vi "Dashboard Main.vi"() -> ()   [LabVIEW 2020]
uses:
  <vilib>/Rock Robotics/Network Tables/NT Read Numeric Array.vi
  <vilib>/Rock Robotics/Network Tables/NT Read String.vi
  <vilib>/Rock Robotics/Network Tables/NT Read Number.vi
  <vilib>/Rock Robotics/Network Tables/NT Read Boolean.vi
  <vilib>/Rock Robotics/Network Tables/NT Write Number.vi
  <vilib>/Rock Robotics/Network Tables/NT Write Boolean.vi
panel:
  out "Popcorn Engaged":bool
  out "Camera Image 5":T1(plugin-control)
  in  "Camera Settings Right":T2={"Frame Rate"=30, "Compression"=30, "Size"=1, "DB Camera Config"=FALSE} {"Frame Rate" scale=1.0..30.0; "Compression" scale=100.0..-1.0; "Size" items=["640x480", "320x240", "160x120"]}
  in  "Camera Name Right":string(combo)="No Camera Selection"
  out "Camera Perf":string
  in  "Camera Settings":T2={"Frame Rate"=30, "Compression"=30, "Size"=1, "DB Camera Config"=FALSE} {"Frame Rate" scale=1.0..30.0; "Compression" scale=100.0..-1.0; "Size" items=["640x480", "320x240", "160x120"]}
  in  "TCP":refnum<k5>
  out "Robot IP":string
  in  "Dashboard Tab":T3(tab)
  in  "ARE YOU READY TO RUMBLE":bool
  out "Climb Override":bool
  out "Climbing Stages":sgl(slide) scale=0.0..10.0 scale format="%#_6p"
  out "Lidar":dbl(knob) scale=0.0..10.0
  out "Reverse":bool
  out "Gyro":bool
  out "Drive Mode":string
  in  "Select Auto":string(combo)="Select Autonomous ..."
  out "NT Connection":bool
  out "MotorChart R":cluster{"Numeric":dbl, "Numeric":dbl}(graph)
  out "MotorChart L":cluster{"Numeric":dbl, "Numeric":dbl}(graph)
  out "MotorSliders R":cluster{"MotorSlide1":dbl, "MotorSlide2":dbl} {"MotorSlide2" scale=-1.0..1.0 scale format="%#_2e"; "MotorSlide1" scale=-1.0..1.0 scale format="%#_2e"}
  out "MotorSliders L":cluster{"MotorSlide1":dbl, "MotorSlide2":dbl} {"MotorSlide2" scale=-1.0..1.0 scale format="%#_2e"; "MotorSlide1" scale=-1.0..1.0 scale format="%#_2e"}
  out "JS1 Z":dbl(slide) scale=-1.0..1.0 scale format="%#_2e"
  out "JS1 Graph":cluster{"X":dbl, "Y":dbl}[](graph)
  out "JS1 Buttons":T4
  out "JS2 Z":dbl(slide) scale=-1.0..1.0 scale format="%#_2e"
  out "JS2 Graph":cluster{"X":dbl, "Y":dbl}[](graph)
  out "JS2 Buttons":T4
  out "Mode":T5(ring)=enum."Auto Disabled"
  out "Camera Image Right":T1(plugin-control)
  out "Shooter Speed":cluster{"Shooter Demand":dbl, "Numeric":dbl}(graph)
  out "Shooter Speed":dbl
  in  "Shooter Demand":dbl
  in  "Dashboard Tab 2":T6(tab)
  out "Speed Chart Left":cluster{"Numeric":dbl, "Numeric":dbl}(graph)
  out "Speed Chart Right":cluster{"Numeric":dbl, "Numeric":dbl}(graph)
  in  "Boolean":bool
  out "Right Speed Demand":dbl
  out "Left Speed Demand":dbl
  out "Right Speed":dbl
  out "Left Speed":dbl
  out "Current Filter":T7={"Hue"={110.0, 142.0}, "Saturation"={0.0, 209.6394230769231}, "Value"={0.0, 105.16949152542372}} {"Value" scale=0.0..255.0; "Saturation" scale=0.0..255.0; "Hue" scale=0.0..255.0 scale format="%#_3g"}
  in  "New Filter":T7={"Hue"={110.0, 142.0}, "Saturation"={0.0, 209.6394230769231}, "Value"={0.0, 105.16949152542372}} {"Value" scale=0.0..255.0; "Saturation" scale=0.0..255.0; "Hue" scale=0.0..255.0 scale format="%#_3g"}
  out "Bananas Engaged":bool
  in  "DONUT PRESS":bool
  out "Bandwidth (Mbps)":dbl
  out "FPS":dbl
  in  "Update":bool
  in  "CheckList":i32[](listbox)
  out "Tree":string(tree)
  out "Camera Image":T1(plugin-control)
  out "Background":bool
  in  "Camera Name":string(combo)="No Camera Selection"
  # "HW"
  # "HW"
  # "Drive Motors"
  # "Joysticks"
  # "Front"
  # "Right"
  # "Left"
  # "Back"
  # "Right"
  # "Left"
  # "Speed D"
  # "Speed"
  # "DONUT PRESS"
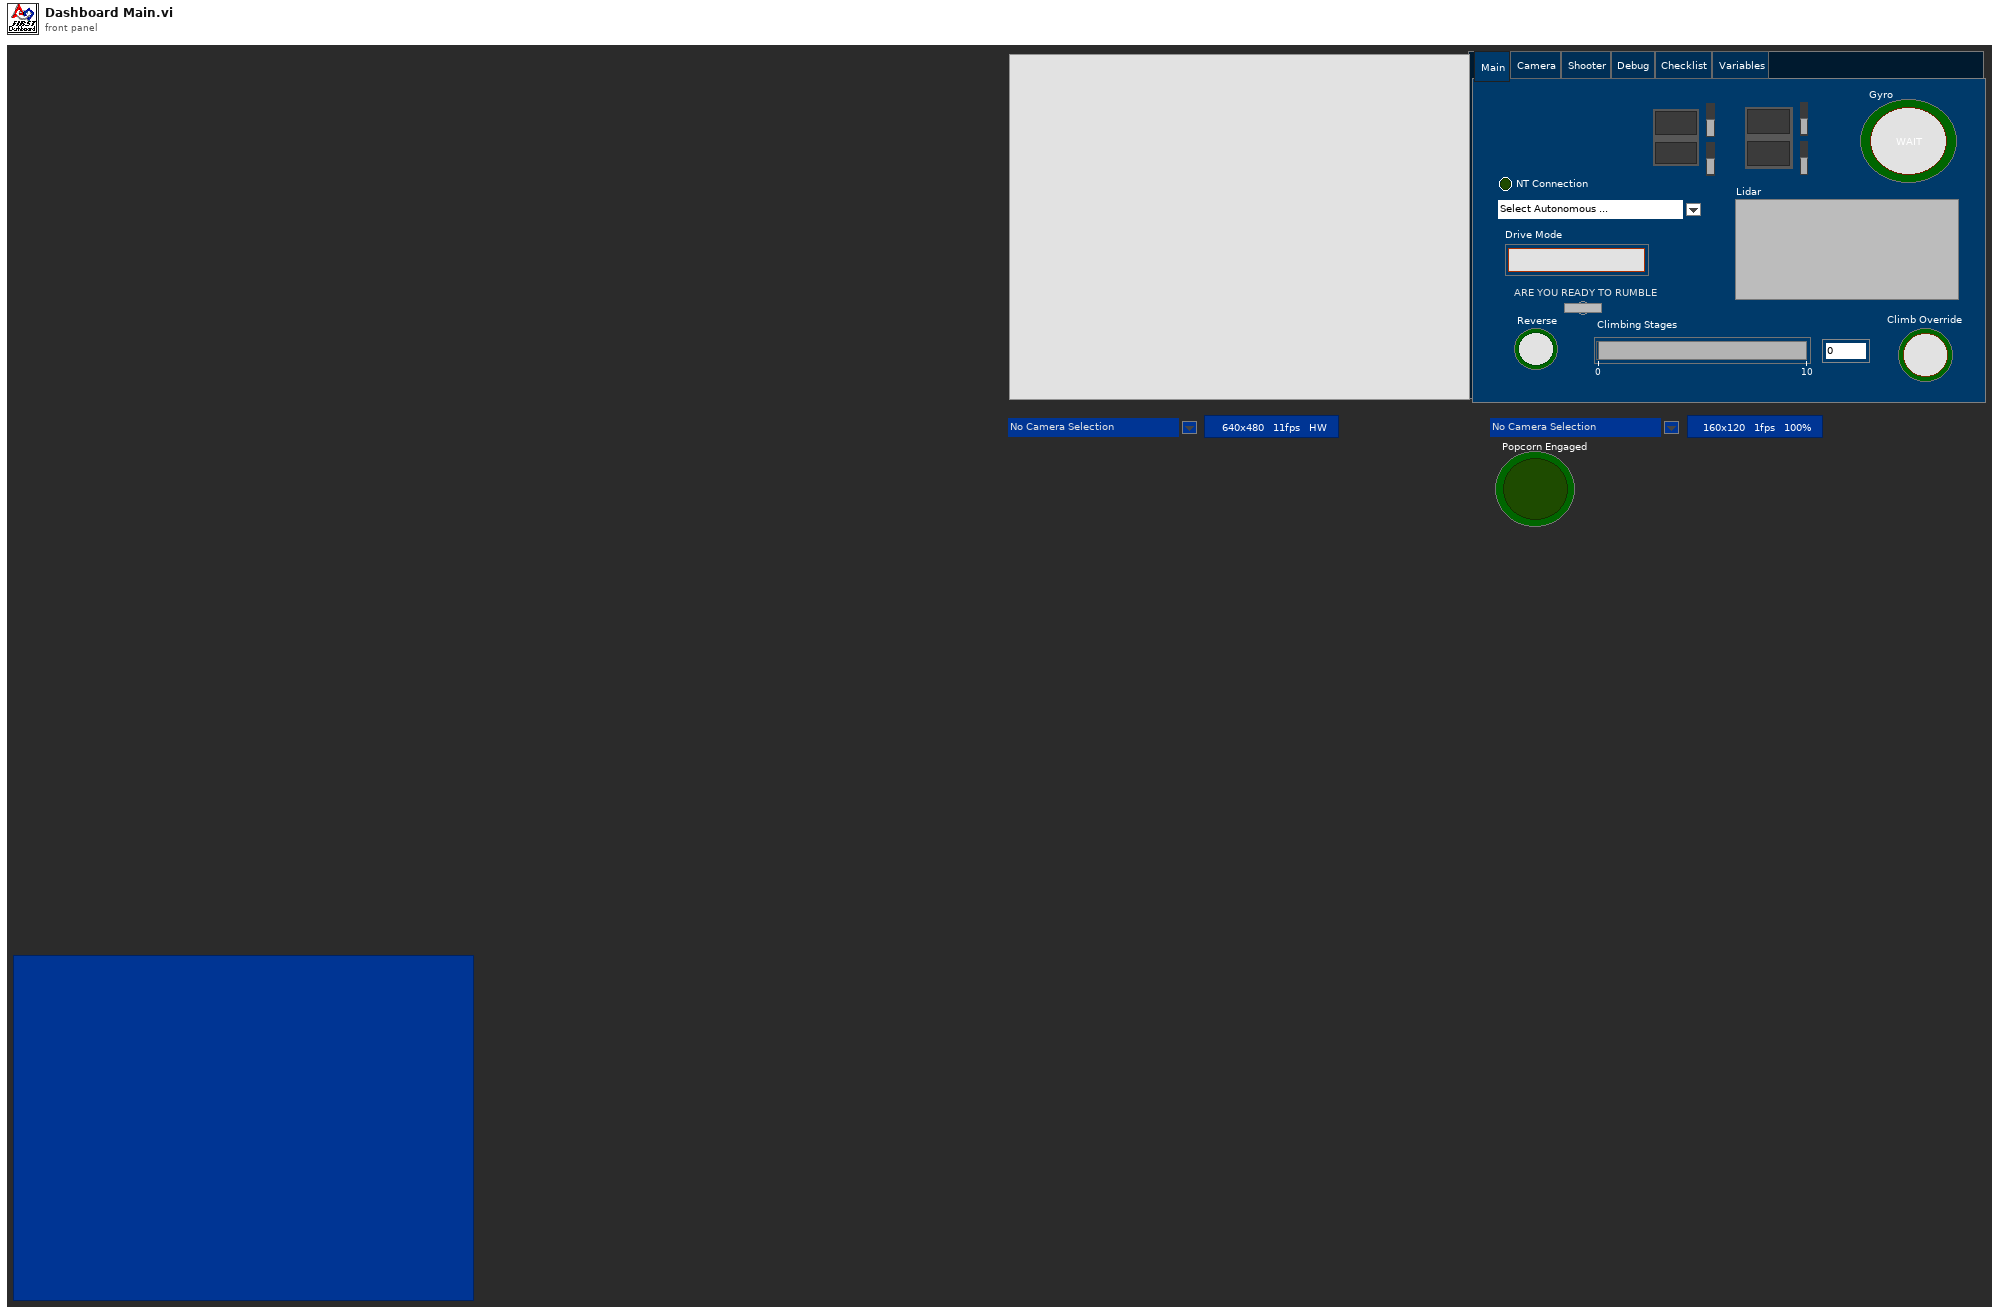
[diagram p1: front panel]
types:
  T1 = typedef "IMAQ Image.ctl" = refnum<image>
  T2 = cluster{"Frame Rate":i32, "Compression":i32, "Size":u16, "DB Camera Config":bool}
  T3 = enum32{"Main", "Camera", "Shooter", "Debug", "Checklist", "Variables"}
  T4 = cluster{bool, bool, bool, bool, bool, bool, bool, bool, bool, bool, bool, bool}
  T5 = enum8{"Tele-Op Disabled", "Tele-Op Enabled", "Auto Disabled", "Auto Enabled", "Test Disabled", "Test Enabled", "Disconnected", "No Code", "E-Stop"}
  T6 = enum32{"Drive Left", "Drive Right", "Table", "Camera", "Random"}
  T7 = cluster{"Hue":cluster{dbl, dbl}, "Saturation":cluster{dbl, dbl}, "Value":cluster{dbl, dbl}}
  T8 = typedef "Image Type" = u32
  T9 = cluster{"Save Path":path, "Interval (s)":dbl, "Keep":i32}
  T10 = cluster{"Camera Image":refnum<vi>, "Dashboard Tab":refnum<vi>, "Background":refnum<vi>, "Tree":refnum<vi>, "Camera Settings":refnum<vi>, "Camera Name":refnum<vi>, "Camera Perf":refnum<vi>}
  T11 = cluster{"Camera Name":string, "Camera File Name":string, "Saved DB Images Info":cluster{"Save Path":path, "Interval (s)":dbl, "Keep":i32}}
  T12 = cluster{cluster{dbl, dbl}, cluster{dbl, dbl}, cluster{dbl, dbl}}
  T13 = cluster{"Shift":bool, "Ctrl":bool, "Alt":bool, "Cmd":bool, "Opt":bool}
  T14 = cluster{"Global Rectangle":i32[], "Contours":cluster{"Contour Type":u32, "ROI Type":u32, "Points":i32[]}[]}
  T15 = cluster{"Camera Name Right":string, string, "Saved DB Images Info":cluster{"Save Path":path, "Interval (s)":dbl, "Keep":i32}}
  T16 = cluster{"Error Strings":string, "Disable Counts":cluster{u16, u16}, "Rail Faults":cluster{u16, u16, u16}, "Robot IP":string, "DB Mode":u8, "Event Info":cluster{"Name":string, "Type":u8, "Number":u16, "Replay":u8}}
  T17 = cluster{"Storage":cluster{"Disk Free":u64, "RAM Block":u32, "RAM free":u32}, "CPU Utilization":cluster{"CPU % ISR":sgl, "CPU % Time Crit":sgl, "CPU % Timed Str":sgl, "CPU % High":sgl, "CPU % Above":sgl, "CPU % Normal":sgl, "CPU % Low":sgl}, "CAN":cluster{"% Bus Utilization":sgl, "Bus Off Cnt":u32, "TX_FIFO Full Cnt":u32, "Receive Error Cnt":u8, "Transmit Error Cnt":u8}, "HID":cluster{"HID Outputs":u32, "Rumble Low":u16, "Rumble High":u16}[]}
  T18 = cluster{"Status bits":cluster{"Test Mode":bool, "Autonomous":bool, "Enabled":bool, "Code Start":bool, "Brownout":bool, "Reserved 2":bool, "Reserved 3":bool, "E-Stop":bool}, "Code Trace":cluster{"Disabled":bool, "TeleOp":bool, "Auto":bool, "Test":bool}, "Controller Type":enum16{"unknown", "cRIO", "roboRio"}, "Code?":enum16{"unknown", "noCode", "code"}, "Battery V":dbl}
  T19 = cluster{"Control Bits":cluster{"TestMode":bool, "Autonomous":bool, "Enabled":bool, "FMS Present":bool, bool, bool, bool, "E-Stop":bool}, "Team Station ":u8, "Countdown":sgl, "Joystick Values":cluster{"Axes":dbl[], "Buttons":bool[], "POVs":i16[]}[]}
  T20 = cluster{"Axes":dbl[], "Buttons":bool[], "POVs":i16[]}[]
  T21 = cluster{"Axes":dbl[], "Buttons":bool[], "POVs":i16[]}
  T22 = cluster{"Buttons[0]":bool, "Buttons[1]":bool, "Buttons[2]":bool, "Buttons[3]":bool, "Buttons[4]":bool, "Buttons[5]":bool, "Buttons[6]":bool, "Buttons[7]":bool, "Buttons[8]":bool, "Buttons[9]":bool, "Buttons[10]":bool, "Buttons[11]":bool}
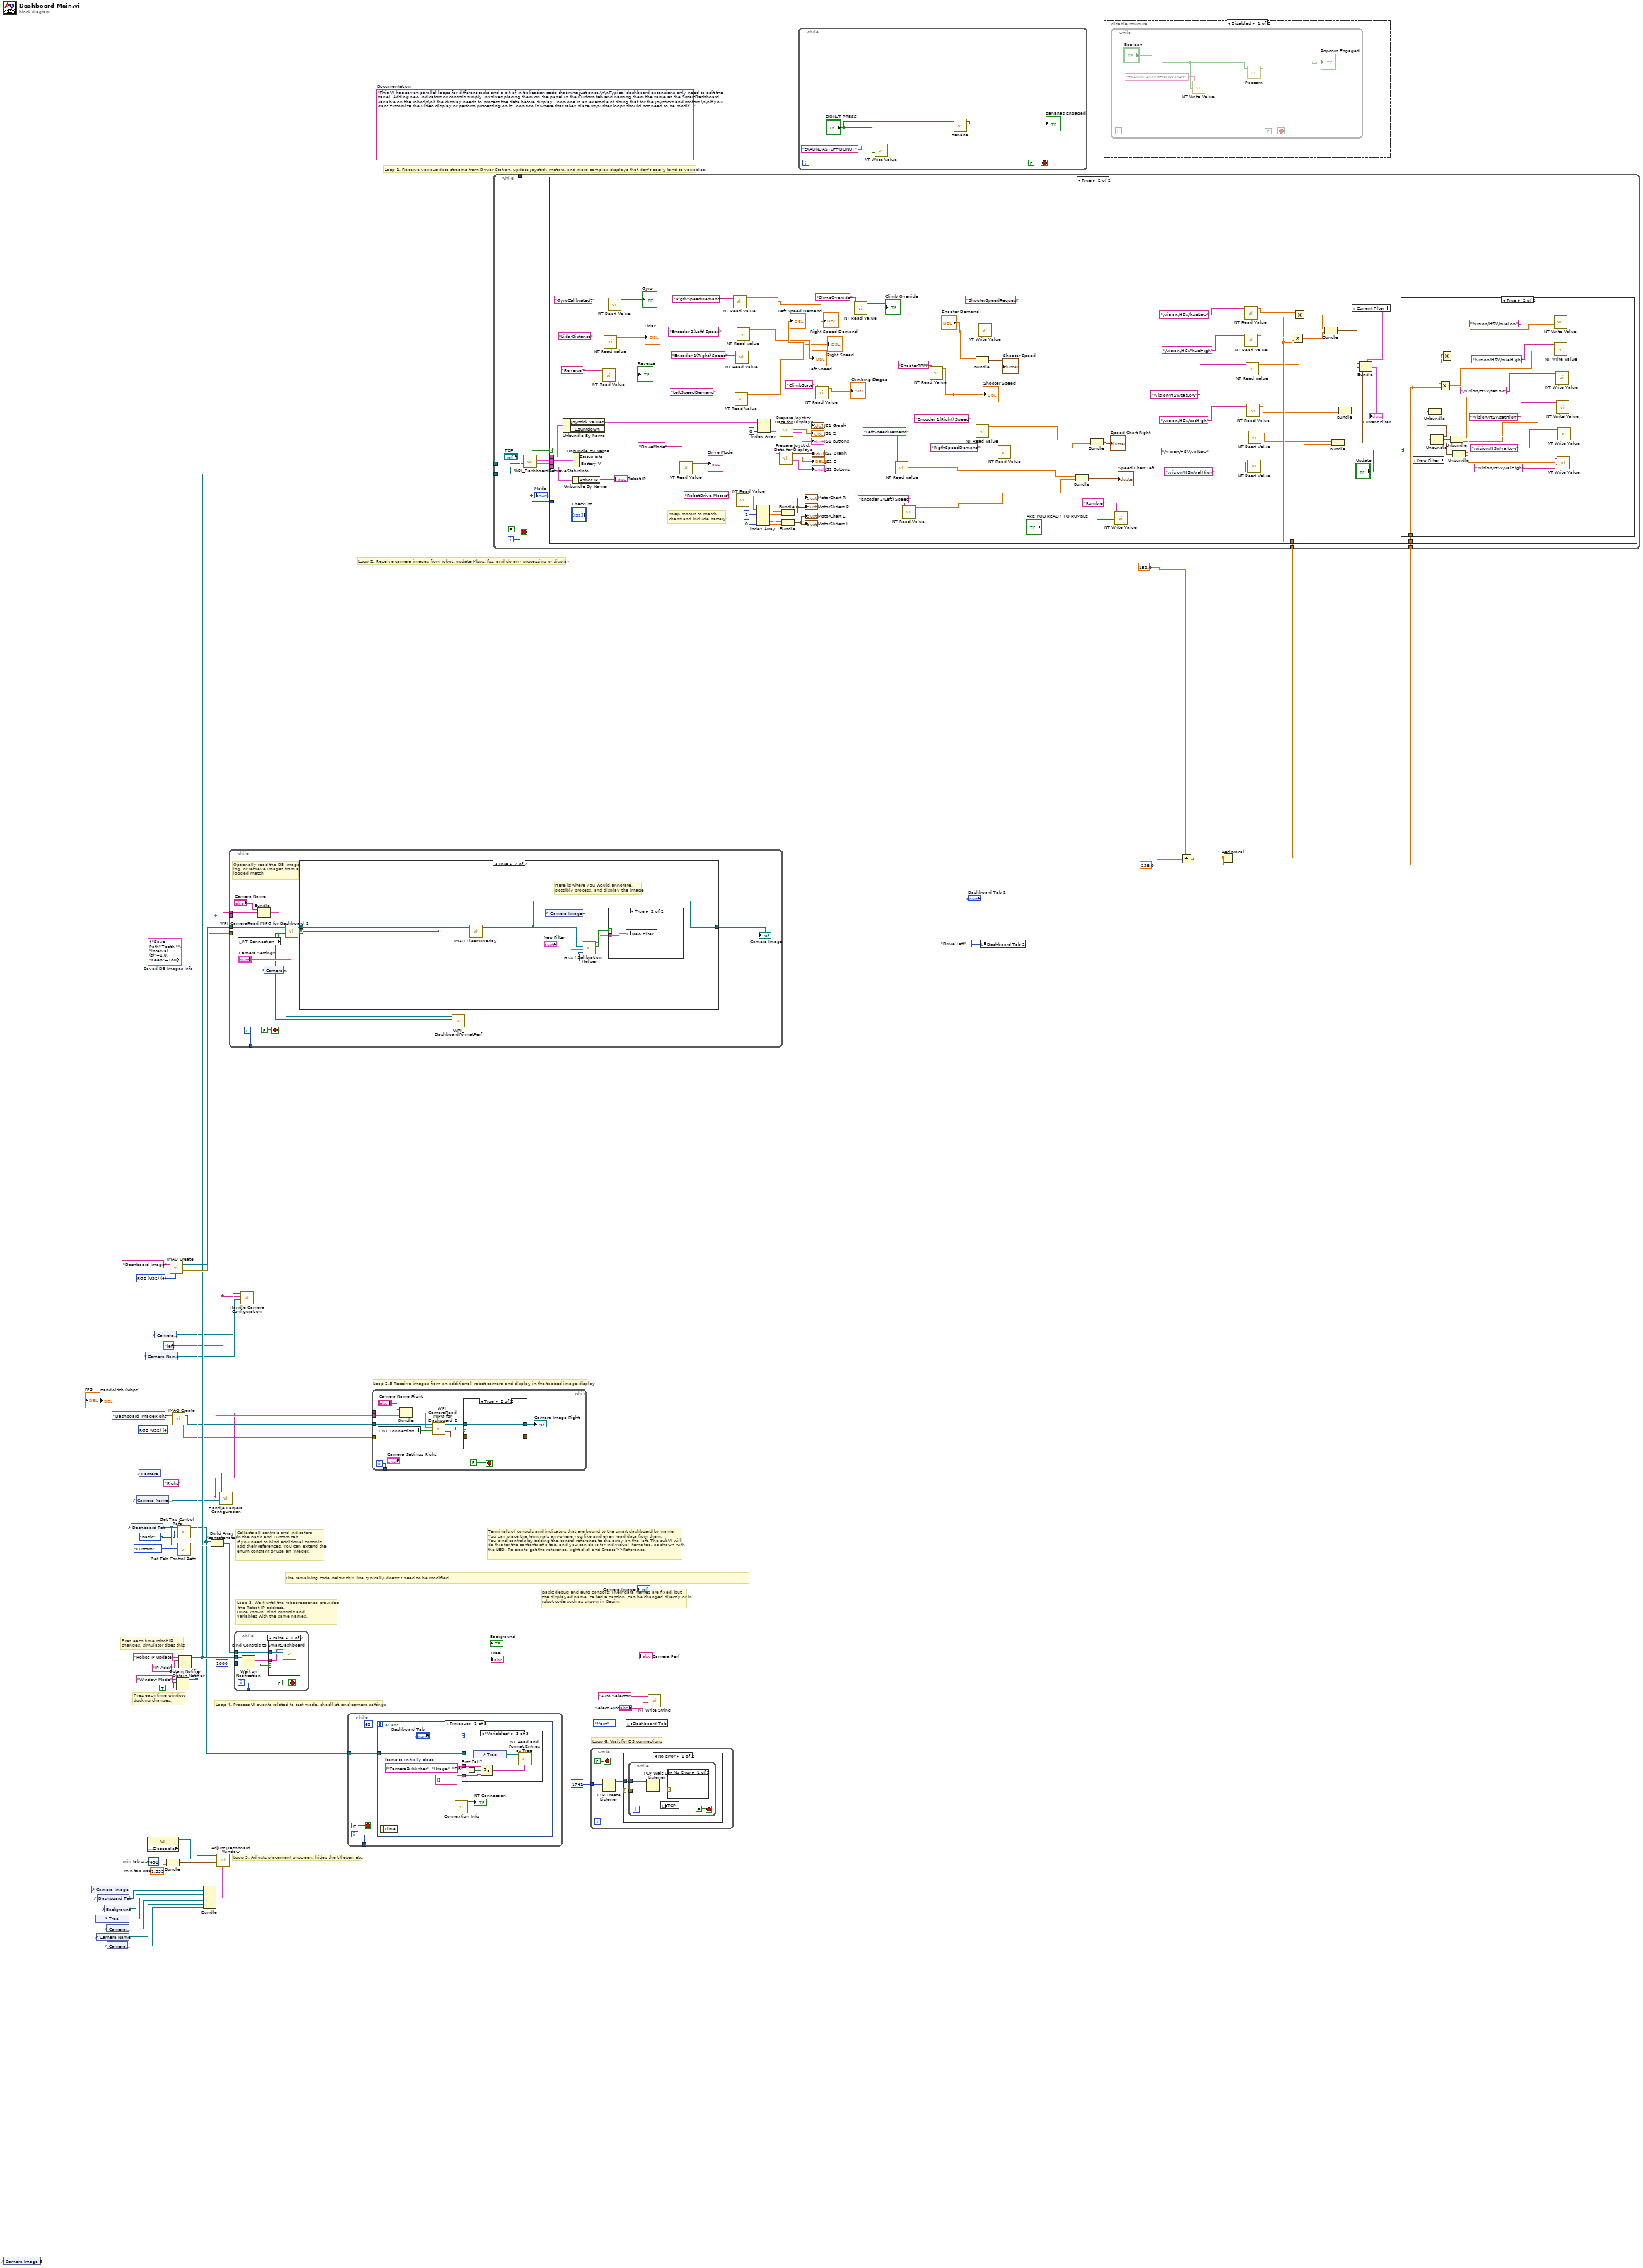
[diagram p0: block diagram]
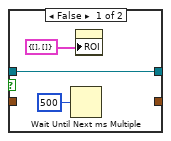
[diagram p3: hidden frame]
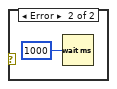
[diagram p4: hidden frame]
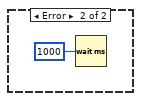
[diagram p5: hidden frame]
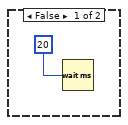
[diagram p6: hidden frame]
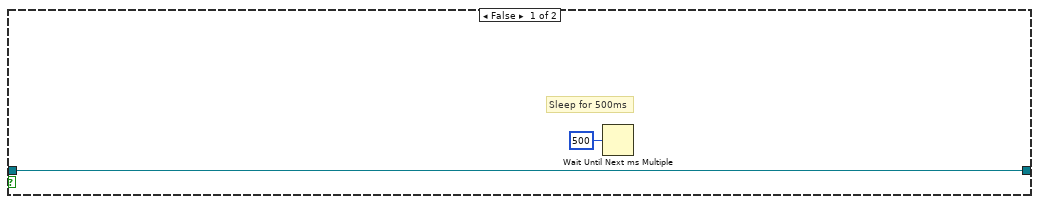
[diagram p9: hidden frame]
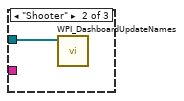
[diagram p12: hidden frame]
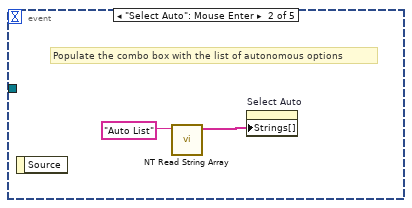
[diagram p13: hidden frame]
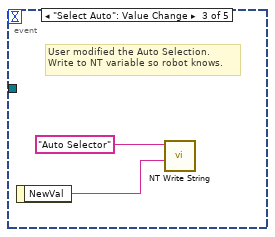
[diagram p14: hidden frame]
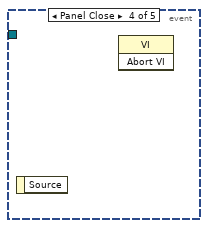
[diagram p15: hidden frame]
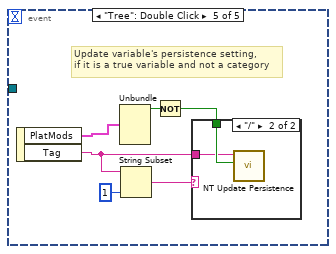
[diagram p16: hidden frame]
diagram:
  w8 = T8 4 items=["Grayscale (U8)", "Grayscale (I16)", "Grayscale (SGL)", "Complex (CSG)", "RGB (U32)", "HSL (U32)", "RGB (U64)"] ("Image Type")
  w10 = "Right"
  w14 = "left" ("Camera File Name")
  w13 = T9 {"Save Path"=path "", "Interval (s)"=1.0, "Keep"=180}  # Saved DB Images Info
  w34 = 491  # min tab size
  w33 = 1.333  # min tab size
  (unwired) "This VI has seven parallel loops for different tasks and a bit of initialization code that runs just once.\n\nTypical dashboard extensions only need to edit the panel. Adding new indicators or controls simply involves placing them on the panel in the Custom tab and naming them the same as the SmartDashboard variable on the robot\n\nIf the display needs to process the data before display, loop one is an example of doing that for the joysticks and motors.\n\nIf you want customize the video display or perform processing on it, loop two is where that takes place.\n\nOther loops should not need to be modified. They are pretty standard, and document the task they perform."  # Documentation
  w49 = T8 4 items=["Grayscale (U8)", "Grayscale (I16)", "Grayscale (SGL)", "Complex (CSG)", "RGB (U32)", "HSL (U32)", "RGB (U64)"] ("Image Type")
  # "Loop 2.5 Receive images from an additional  robot camera and display in the tabbed image display"
  # "Loop 6. Wait for DS connections"
  # "Basic debug and auto controls: Their data names are fixed, but\nthe displayed name, called a caption, can be changed directly or in\nrobot code such as shown in Begin."
  # "Fires each time robot IP\nchanges, simulator does this"
  # "Fires each time window\ndocking changes."
  # "Collects all controls and indicators\nin the Basic and Custom tab.\nIf you need to bind additional controls,\nadd their references. You can extend the\nenum constant or use an integer."
  # "The remaining code below this line typically doesn't need to be modified."
  # "Loop 4. Process UI events related to test mode, checklist, and camera settings"
  # "Terminals of controls and indicators that are bound to the smart dashboard by name.\nYou can place the terminals anywhere you like and even read data from them.\nYou bind controls by adding the control reference to the array on the left. The subVI will\ndo this for the contents of a tab, and you can do it for individual items too, as shown with\nthe LED. To create get the reference, right-click and Create>>Reference."
  # "Loop 3. Wait until the robot response provides\n the Robot IP address.\nOnce known, bind controls and\nvariables with the same names."
  # "Loop 5. Adjusts placement onscreen, hides the titlebar, etc."
  # "Loop 1. Receive various data streams from Driver Station, update joystick, motors, and more complex displays that don't easily bind to variables."
  # "Loop 2. Receive camera images from robot, update Mbps, fps, and do any processing or display"
  n1 = control-ref of="Camera Image 5"() -> ()  [unwired: 1 out]
  n2 = control-ref of="Camera Image"() -> (w36:refnum<vi>)
  n3 = control-ref of="Tree"() -> (w20:refnum<vi>)
  n4 = control-ref of="Camera Name"() -> (w18:refnum<vi>)
  n5 = control-ref of="Dashboard Tab"() -> (w35:refnum<vi>)
  n6 = control-ref of="Background"() -> (w31:refnum<vi>)
  n7 = control-ref of="Camera Settings"() -> (w19:refnum<vi>)
  n8 = control-ref of="Camera Perf"() -> (w17:refnum<vi>)
  n9 = control-ref of="Dashboard Tab"() -> (w39:refnum<vi>)
  n10 = control-ref of="Camera Name Right"() -> (w11:refnum<vi>)
  n11 = control-ref of="Camera Settings Right"() -> (w12:refnum<vi>)
  n12 = control-ref of="Camera Name"() -> (w24:refnum<vi>)
  n13 = property class="VI" props=["Front Panel.Closeable"]() -> (reference out=w40:refnum<vi>)  [unwired: 2 in, 2 out]
  n14 = control-ref of="Camera Settings"() -> (w25:refnum<vi>)
  n15 = Bundle("min tab size"=w34, "min tab size"=w33) -> (w32:cluster{"min tab size":i32, "min tab size":dbl})  [unwired: 1 in]
  n16 = call "IMAQ Create"("Image Name"="Dashboard Image", "Image Type"=w49) -> ("New Image"=w47:T1, "error out"=w46:errorcluster)  [unwired: 2 in, 1 out]
  n17 = call "IMAQ Create"("Image Name"="Dashboard ImageRight", "Image Type"=w8) -> ("New Image"=w7:T1, "error out"=w6:errorcluster)  [unwired: 2 in, 1 out]
  n18 = Obtain Notifier(name (unnamed)="Window Mode", notification data type=TRUE) -> (notifier out=w28:refnum<notifier>)  [unwired: 2 in, 2 out]
  n19 = call <vilib>:"Get Tab Control Refs.vi"("Page Index"=enum32{"Drive", "Basic", "Custom", "Variables"}."Basic" ("Dashboard Tab"), "TabControl in"=w39) -> ("ControlsOnPage"=w23:refnum<vi>[])  [unwired: 9 in]
  n20 = call <vilib>:"Get Tab Control Refs.vi"("Page Index"=enum32{"Drive", "Basic", "Custom", "Variables"}."Custom" ("Dashboard Tab"), "TabControl in"=w39) -> ("ControlsOnPage"=w38:refnum<vi>[])  [unwired: 9 in]
  n21 = Obtain Notifier(name (unnamed)="Robot IP Update", notification data type="IP Addr" ("name (unnamed)")) -> (notifier out=w29:refnum<notifier>)  [unwired: 2 in, 2 out]
  n22 = Bundle("Camera Image"=w36, "Dashboard Tab"=w35, "Background"=w31, "Tree"=w20, "Camera Settings"=w19, "Camera Name"=w18, "Camera Perf"=w17) -> (w30:T10)  [unwired: 1 in]
  n23 = Build Array (concatenate)(w23, w38) -> (w37:refnum<vi>[])
  n24 = call "Adjust Dashboard Window.vi"("Sizing Refnums"=w30, "Size Constraints"=w32, "VI"=w40, "WIn Mode"=w28) -> ()  [unwired: 8 in]
  n25 = call "Handle Camera Configuration.vi"("CameraNameRef"=w11, "Display Name"=w10, "ClusterRef"=w12) -> ()  [unwired: 9 in]
  n26 = while {
    tunnel: w47 -> [w61]
    tunnel: w46 -> [_]
    tunnel: [w62] -> _
    tunnel: w13 -> [w55]
    tunnel: w14 -> [w52]
    i -> [w62]
    stop <- FALSE stop-if-true
    # "Optionally read the DB image,\nlog, or retrieve images from a\nlogged match"
    n27 = local read "NT Connection"() -> (w56:bool)
    n28 = Bundle("Camera Name"="Camera Name", "Camera File Name"=w52, "Saved DB Images Info"=w55) -> (w54:T11)  [unwired: 1 in]
    n29 = control-ref of="Camera Perf"() -> (w50:refnum<vi>)
    n30 = call <vilib>:"WPI_CameraRead MJPG for Dashboard_2.vi"("Camera Settings"="Camera Settings", "NT Connection"=w56, "Capture Info"=w54, "Image in"=w61) -> ("perf info"=w51:cluster{"Bandwidth (Mbps)":dbl, "fps":dbl}, "Active"=w59:bool, "Image\\ out"=w60:T1)  [unwired: 5 in]
    n31 = case shown="True" w59 {
      tunnel: w60 -> [w64 w72]
      tunnel: [w64 w70] -> w57
      frame False {
        # "Sleep for 500ms"
        n32 = Wait Until Next ms Multiple(millisecond multiple=u32 500) -> ()  [unwired: 1 out]
      }
      frame True {
        w67 = u16 2 items=["RGB", "HSL", "HSV", "HSI", "CIE L*a*b*", "CIE XYZ"] ("Color Mode")
        # "Here is where you would annotate,\npossibly process, and display the image"
        n33 = call "IMAQ Clear Overlay"("Image"=w72) -> ("Image Out"=w70:T1)  [unwired: 2 in, 8 out]
        n34 = control-ref of="Camera Image"() -> (w66:refnum<vi>)
        n35 = call "Calibration Helper.vi"("Color Mode"=w67, "Color Components"="New Filter", "Image"=w70, "Image Ctl Refnum"=w66) -> ("Changed"=w69:bool, "output color"=w68:T12)  [unwired: 6 in]
        n36 = case shown="True" w69 {
          tunnel: w68 -> [_ w73]
          frame False {
          }
          frame True {
            n37 = local write "New Filter"(w73) -> ()
          }
        }
      }
    }
    "Camera Image" <- w57
    n38 = call <vilib>:"WPI_DashboardFormatPerf.vi"("Performance"=w51, "String in"=w50) -> ()  [unwired: 10 in]
  }
  n39 = while {
    tunnel: w37 -> [w80]
    tunnel: w29 -> [w78]
    tunnel: [w76] -> _
    tunnel: u32 1000 ("milliseconds to wait") -> [w75]
    i -> [w76]
    stop <- FALSE stop-if-true
    n40 = Wait on Notification(notifier=w78, timeout in ms (-1)=w75) -> (notification=w77:string, timed out?=w74:bool)  [unwired: 2 in, 2 out]
    n41 = case shown="False" w74 {
      tunnel: w80 -> [w82 _]
      tunnel: w77 -> [w81 _]
      frame False {
        n42 = call <vilib>:"Bind Controls to SmartDashboard.vi"("Bound Control Refs"=w82, "Server IP Address"=w81) -> ()  [unwired: 10 in]
      }
      frame True {
      }
    }
  }
  n43 = call "Handle Camera Configuration.vi"("CameraNameRef"=w24, "Display Name"=w14, "ClusterRef"=w25) -> ()  [unwired: 9 in]
  n44 = while {
    tunnel: [w84] -> _
    tunnel: w23 -> [w83]
    i -> [w84]
    stop <- FALSE stop-if-true
    n45 = event shown="[0] Timeout" {
      selector: _ -> [_ _ _ _ _]
      dyn-events: _ -> [_ _ _ _ _]
      timeout: u32 60 ("milliseconds to wait") -> [_ _ _ _ _]
      tunnel: w83 -> [w89 _ _ _ _]
      event Timeout {
        w88 = string[] ["CameraPublisher", "Usage", "DB"]  # Items to initially close
        n46 = event-data() -> ()  [unwired: 1 in, 1 out]
        n47 = call <vilib>:"Connextion Info.vi"() -> ("Connected"=→"NT Connection":bool)  [unwired: 10 in, 1 out]
        n48 = case shown="\"Variables\"" "Dashboard Tab" {
          tunnel: w89 -> [_ w92 _]
          tunnel: w88 -> [_ _ w95]
          tunnel: string[] [] -> [_ _ w94]
          frame "Debug", Default {
          }
          frame "Shooter" {
            n49 = call <vilib>:"WPI_DashboardUpdateNames.vi"("Controls on Tab"=w92) -> ()  [unwired: 11 in]
          }
          frame "Variables" {
            n50 = First Call?() -> (First Call?: T/F=w96:bool)
            n51 = control-ref of="Tree"() -> (w97:refnum<vi>)
            n52 = Select(t=w95, s=w96, f=w94) -> (s? t:f=w93:string[])
            n53 = call <vilib>:"NT Read and Format Entries as Tree.vi"("Tags to  Close"=w93, "Tree Refnum"=w97) -> ()  [unwired: 8 in, 2 out]
          }
        }
      }
      event "Select Auto": Mouse Enter {
        # "Populate the combo box with the list of autonomous options"
        n54 = event-data() -> ()  [unwired: 1 in, 1 out]
        n55 = call <vilib>:"NT Read String Array.vi"("Name"="Auto List") -> ("String Array"=w98:string[])  [unwired: 9 in, 1 out]
        n56 = property on="Select Auto" class="CmbBox"("Strings[]"=w98) -> ()  [unwired: 2 in, 2 out]
      }
      event "Select Auto": Value Change {
        # "User modified the Auto Selection.\nWrite to NT variable so robot knows."
        n57 = event-data() -> ("NewVal"=w100:string)  [unwired: 1 in]
        n58 = call <vilib>:"NT Write String.vi"("String"=w100, "Name"="Auto Selector") -> ()  [unwired: 9 in, 1 out]
      }
      event Panel Close {
        n59 = event-data() -> ()  [unwired: 1 in, 1 out]
        n60 = invoke class="VI" method="Abort VI"() -> ()  [unwired: 3 in, 3 out]
      }
      event "Tree": Double Click {
        # "Update variable's persistence setting,\nif it is a true variable and not a category"
        n61 = event-data() -> ("PlatMods"=w103:T13, "Tag"=w102:string)  [unwired: 1 in]
        n62 = Unbundle(w103) -> ("Shift"=w107:bool)  [unwired: 4 out]
        n63 = String Subset(string=w102, length (rest)=1 ("length (rest)")) -> (substring=w104:string)  [unwired: 1 in]
        n64 = Not(x=w107) -> (.not. x?=w106:bool)
        n65 = case shown="\"/\"" w104 {
          tunnel: w106 -> [_ w109]
          tunnel: w102 -> [_ w108]
          frame Default {
          }
          frame "/" {
            n66 = call <vilib>:"NT Update Persistence.vi"("Persistence"=w109, "Name"=w108) -> ()  [unwired: 9 in, 1 out]
          }
        }
      }
    }
  }
  n67 = while {
    tunnel: w7 -> [w122]
    tunnel: [w118] -> _
    tunnel: w13 -> [w114]
    tunnel: w10 -> [w111]
    tunnel: w6 -> [_]
    i -> [w118]
    stop <- FALSE stop-if-true
    n68 = local read "NT Connection"() -> (w115:bool)
    n69 = Bundle("Camera Name Right"="Camera Name Right", w111, "Saved DB Images Info"=w114) -> (w113:T15)  [unwired: 1 in]
    n70 = call <vilib>:"WPI_CameraRead MJPG for Dashboard_2.vi"("Camera Settings"="Camera Settings Right", "NT Connection"=w115, "Capture Info"=w113, "Image in"=w122) -> ("perf info"=w110:cluster{"Bandwidth (Mbps)":dbl, "fps":dbl}, "Active"=w117:bool, "Image\\ out"=w120:T1)  [unwired: 5 in]
    n71 = case shown="True" w117 {
      tunnel: w120 -> [w124 w127]
      tunnel: [w124 w127] -> w116
      tunnel: [_ w126] -> _
      tunnel: w110 -> [_ w126]
      frame False {
        n72 = Wait Until Next ms Multiple(millisecond multiple=u32 500) -> ()  [unwired: 1 out]
        n73 = property on="Camera Image Right" class="ImageControl"("ROI"=T14 {"Global Rectangle"=[], "Contours"=[]}) -> ()  [unwired: 2 in, 2 out]
      }
      frame True {
      }
    }
    "Camera Image Right" <- w116
  }
  n74 = while {
    tunnel: u16 1741 ("timeout ms (25000)") -> [w129]
    stop <- FALSE stop-if-true
    n75 = TCP Create Listener(10:w129) -> (0:w128:errorcluster, 3:w130:refnum<k5>)  [unwired: 4 in, 1 out]
    n76 = case shown="No Error" w128 {
      selector: w128 -> [w132 _]
      tunnel: w130 -> [w133 _]
      frame No Error {
        n77 = while {
          tunnel: w133 -> [w136]
          tunnel: w132 -> [w135]
          stop <- FALSE stop-if-true
          n78 = TCP Wait On Listener(8:w135, 11:w136) -> (0:w137:errorcluster, 4:w138:refnum<k5>)  [unwired: 2 in, 3 out]
          n79 = local write "TCP"(w138) -> ()
          n80 = case shown="No Error" w137 {
            frame No Error {
            }
            frame Error {
              n81 = Wait (ms)(milliseconds to wait=u32 1000) -> ()  [unwired: 1 out]
            }
          }
        }
      }
      frame Error {
        n82 = Wait (ms)(milliseconds to wait=u32 1000) -> ()  [unwired: 1 out]
      }
    }
  }
  n83 = local write "Dashboard Tab"(T3."Main" ("Dashboard Tab")) -> ()
  n84 = call <vilib>:"NT Write String.vi"("String"="Select Auto", "Name"="Auto Selector") -> ()  [unwired: 9 in, 1 out]
  n85 = while {
    stop <- FALSE stop-if-true
    n86 = call-poly <vilib>:"NT Write Value.vi"("Boolean"="DONUT PRESS", "Name"="zKALINDASTUFF/DONUT") -> ()  [unwired: 9 in, 1 out]
    n87 = call "Banana.vi"("Boolean"="DONUT PRESS") -> ("Boolean 2"=→"Bananas Engaged":bool)  [unwired: 10 in]
  }
  n88 = local write "Dashboard Tab 2"(T6."Drive Left" ("Dashboard Tab")) -> ()
  n89 = disable-structure shown="Disabled" {
    frame Disabled {
      n90 = while {
        stop <- FALSE stop-if-true
        n91 = call-poly <vilib>:"NT Write Value.vi"("Boolean"="Boolean", "Name"="zKALINDASTUFF/POPCORN") -> ()  [unwired: 9 in, 1 out]
        n92 = call "Popcorn.vi"("Boolean"="Boolean") -> ("Boolean 2"=→"Popcorn Engaged":bool)  [unwired: 10 in]
      }
    }
    frame Enabled {
    }
  }
  n93 = Divide(x=180.0, y=256.0) -> (x/y=w1:dbl)
  n94 = Reciprocal(x=w1) -> (1/x=w2:dbl)
  n95 = while {
    tunnel: [w160] -> _
    tunnel: w29 -> [w154]
    tunnel: w28 -> [w151]
    tunnel: w2 -> [w150]
    tunnel: w1 -> [w149]
    i -> [w160]
    stop <- FALSE stop-if-true
    n96 = call <vilib>:"WPI_DashboardRetrieveStatusInfo.vi"("Binding Refnum"=w154, "Window Mode Notifier"=w151, "TCP Cnx"="TCP") -> ("Power and Errors"=w155:T16, "Robot Metrics"=w158:T17, "Status Info"=w159:T18, "Control Info"=w156:T19, "Robot Mode"=w153:T5, "Process?"=w157:bool)  [unwired: 3 in]
    "Mode" <- w153
    n97 = case shown="True" w157 {
      tunnel: w159 -> [_ w245]
      tunnel: w158 -> [_ _]
      tunnel: w156 -> [_ w244]
      tunnel: w155 -> [_ w243]
      tunnel: w153 -> [_ _]
      tunnel: w150 -> [_ w182]
      tunnel: w149 -> [_ w171]
      frame False {
        n98 = Wait (ms)(milliseconds to wait=u32 20) -> ()  [unwired: 1 out]
      }
      frame True {
        # "swap motors to match\ncharts and include battery"
        n99 = Unbundle By Name(w244) -> ("Joystick Values"=w234:T20)  [unwired: 1 out]
        n100 = Unbundle By Name(w243) -> ("Robot IP"=→"Robot IP":string)
        n101 = Unbundle By Name(w245) -> ()  [unwired: 2 out]
        n102 = call-poly <vilib>:"NT Read Value.vi"("Name"="Reverse?") -> ("Boolean"=→"Reverse":bool)  [unwired: 9 in, 1 out]
        n103 = call-poly <vilib>:"NT Read Value.vi"("Name"="LidarDistance") -> ("Numeric"=→"Lidar":dbl)  [unwired: 9 in, 1 out]
        n104 = call-poly <vilib>:"NT Read Value.vi"("Name"="GyroCalibrated?") -> ("Boolean"=→"Gyro":bool)  [unwired: 9 in, 1 out]
        n105 = call-poly <vilib>:"NT Read Value.vi"("Name"="DriveMode") -> ("String"=→"Drive Mode":string)  [unwired: 9 in, 1 out]
        n106 = call-poly <vilib>:"NT Read Value.vi"("Name"="RigthSpeedDemand") -> ("Numeric"=→"Right Speed Demand":dbl)  [unwired: 9 in, 1 out]
        n107 = call-poly <vilib>:"NT Read Value.vi"("Name"="LeftSpeedDemand") -> ("Numeric"=→"Left Speed Demand":dbl)  [unwired: 9 in, 1 out]
        n108 = call-poly <vilib>:"NT Read Value.vi"("Name"="Encoder 1(Right) Speed") -> ("Numeric"=→"Right Speed":dbl)  [unwired: 9 in, 1 out]
        n109 = call-poly <vilib>:"NT Read Value.vi"("Name"="RobotDrive Motors") -> ("Numeric Array"=w224:dbl[])  [unwired: 9 in, 1 out]
        n110 = call-poly <vilib>:"NT Read Value.vi"("Name"="Encoder 2(Left) Speed") -> ("Numeric"=→"Left Speed":dbl)  [unwired: 9 in, 1 out]
        n111 = Index Array(array=w224, index #1=1, index #4=0) -> (element #1=w238:dbl, element #2=w239:dbl, element #3=w237:dbl, element #4=w242:dbl)  [unwired: 2 in]
        n112 = Index Array(array=w234, index #2=0 ("index")) -> (element #1=w233:T21, element #2=w229:T21)  [unwired: 1 in]
        n113 = call "Prepare Joystick Data for Displays.vi"("Joystick Values"=w229) -> ("Buttons"=→"JS2 Buttons":T22, "Z Axis"=→"JS2 Z":dbl, "Cartesian Data"=→"JS2 Graph":cluster{"X axis":dbl, "X axis":dbl}[])  [unwired: 8 in]
        n114 = call "Prepare Joystick Data for Displays.vi"("Joystick Values"=w233) -> ("Buttons"=→"JS1 Buttons":T22, "Z Axis"=→"JS1 Z":dbl, "Cartesian Data"=→"JS1 Graph":cluster{"X axis":dbl, "X axis":dbl}[])  [unwired: 8 in]
        n115 = Bundle("Numeric"=w237, "Numeric"=w238) -> (→"MotorChart R" →"MotorSliders R":cluster{"Numeric":dbl, "Numeric":dbl})  [unwired: 1 in]
        n116 = Bundle("Numeric"=w239, "Numeric"=w242) -> (→"MotorChart L" →"MotorSliders L":cluster{"Numeric":dbl, "Numeric":dbl})  [unwired: 1 in]
        n117 = call-poly <vilib>:"NT Read Value.vi"("Name"="ClimbState") -> ("Numeric"=→"Climbing Stages":dbl)  [unwired: 9 in, 1 out]
        n118 = call-poly <vilib>:"NT Read Value.vi"("Name"="ClimbOverride") -> ("Boolean"=→"Climb Override":bool)  [unwired: 9 in, 1 out]
        n119 = call-poly <vilib>:"NT Read Value.vi"("Name"="LeftSpeedDemand") -> ("Numeric"=w216:dbl)  [unwired: 9 in, 1 out]
        n120 = call-poly <vilib>:"NT Read Value.vi"("Name"="Encoder 2(Left) Speed") -> ("Numeric"=w215:dbl)  [unwired: 9 in, 1 out]
        n121 = call-poly <vilib>:"NT Read Value.vi"("Name"="ShooterRPM") -> ("Numeric"=w192:dbl)  [unwired: 9 in, 1 out]
        "Shooter Speed" <- w192
        n122 = Bundle("Shooter Demand"="Shooter Demand", "Numeric"=w192) -> (→"Shooter Speed":cluster{"Shooter Demand":dbl, "Numeric":dbl})  [unwired: 1 in]
        n123 = call-poly <vilib>:"NT Read Value.vi"("Name"="Encoder 1(Right) Speed") -> ("Numeric"=w214:dbl)  [unwired: 9 in, 1 out]
        n124 = call-poly <vilib>:"NT Write Value.vi"("Numeric"="Shooter Demand", "Name"="ShooterSpeedRequest") -> ()  [unwired: 9 in, 1 out]
        n125 = call-poly <vilib>:"NT Read Value.vi"("Name"="RigthSpeedDemand") -> ("Numeric"=w213:dbl)  [unwired: 9 in, 1 out]
        n126 = Bundle("Numeric"=w216, "Numeric"=w215) -> (→"Speed Chart Left":cluster{"Numeric":dbl, "Numeric":dbl})  [unwired: 1 in]
        n127 = Bundle("Numeric"=w214, "Numeric"=w213) -> (→"Speed Chart Right":cluster{"Numeric":dbl, "Numeric":dbl})  [unwired: 1 in]
        n128 = call-poly <vilib>:"NT Write Value.vi"("Boolean"="ARE YOU READY TO RUMBLE", "Name"="Rumble") -> ()  [unwired: 9 in, 1 out]
        n129 = call-poly <vilib>:"NT Read Value.vi"("Name"="/vision/HSV/hueLow") -> ("Numeric"=w184:dbl)  [unwired: 9 in, 1 out]
        n130 = call-poly <vilib>:"NT Read Value.vi"("Name"="/vision/HSV/hueHigh") -> ("Numeric"=w183:dbl)  [unwired: 9 in, 1 out]
        n131 = call-poly <vilib>:"NT Read Value.vi"("Name"="/vision/HSV/satLow") -> ("Numeric"=w179:dbl)  [unwired: 9 in, 1 out]
        n132 = call-poly <vilib>:"NT Read Value.vi"("Name"="/vision/HSV/satHigh") -> ("Numeric"=w178:dbl)  [unwired: 9 in, 1 out]
        n133 = call-poly <vilib>:"NT Read Value.vi"("Name"="/vision/HSV/valHigh") -> ("Numeric"=w176:dbl)  [unwired: 9 in, 1 out]
        n134 = call-poly <vilib>:"NT Read Value.vi"("Name"="/vision/HSV/valLow") -> ("Numeric"=w177:dbl)  [unwired: 9 in, 1 out]
        n135 = Multiply(x=w183, y=w182) -> (x*y=w180:dbl)
        n136 = Multiply(x=w184, y=w182) -> (x*y=w181:dbl)
        n137 = Bundle(w181, w180) -> (w175:cluster{dbl, dbl})  [unwired: 1 in]
        n138 = Bundle("Numeric"=w177, "Numeric"=w176) -> (w173:cluster{"Numeric":dbl, "Numeric":dbl})  [unwired: 1 in]
        n139 = Bundle("Numeric"=w179, "Numeric"=w178) -> (w174:cluster{"Numeric":dbl, "Numeric":dbl})  [unwired: 1 in]
        n140 = local read "Current Filter"() -> (w170:T7)
        n141 = Bundle(cluster=w170, "Hue"=w175, "Saturation"=w174, "Value"=w173) -> (→"Current Filter":T7)
        n142 = case shown="True" "Update" {
          tunnel: w171 -> [_ w257]
          frame False {
          }
          frame True {
            n143 = local read "New Filter"() -> (w258:T7)
            n144 = Unbundle(w258) -> ("Hue"=w256:cluster{dbl, dbl}, "Saturation"=w251:cluster{dbl, dbl}, "Value"=w250:cluster{dbl, dbl})
            n145 = Unbundle(w256) -> (w255:dbl, w254:dbl)
            n146 = Multiply(x=w254, y=w257) -> (x*y=w252:dbl)
            n147 = Multiply(x=w255, y=w257) -> (x*y=w253:dbl)
            n148 = Unbundle(w251) -> (w247:dbl, w246:dbl)
            n149 = Unbundle(w250) -> (w249:dbl, w248:dbl)
            n150 = call-poly <vilib>:"NT Write Value.vi"("Numeric"=w253, "Name"="/vision/HSV/hueLow") -> ()  [unwired: 9 in, 1 out]
            n151 = call-poly <vilib>:"NT Write Value.vi"("Numeric"=w252, "Name"="/vision/HSV/hueHigh") -> ()  [unwired: 9 in, 1 out]
            n152 = call-poly <vilib>:"NT Write Value.vi"("Numeric"=w247, "Name"="/vision/HSV/satLow") -> ()  [unwired: 9 in, 1 out]
            n153 = call-poly <vilib>:"NT Write Value.vi"("Numeric"=w246, "Name"="/vision/HSV/satHigh") -> ()  [unwired: 9 in, 1 out]
            n154 = call-poly <vilib>:"NT Write Value.vi"("Numeric"=w248, "Name"="/vision/HSV/valHigh") -> ()  [unwired: 9 in, 1 out]
            n155 = call-poly <vilib>:"NT Write Value.vi"("Numeric"=w249, "Name"="/vision/HSV/valLow") -> ()  [unwired: 9 in, 1 out]
          }
        }
      }
    }
  }
